vi "reprocess channel names for duplicates.vi"(11 "channels in":cluster{"Name":string, "Path":string}[](array[cluster])) -> (3 "processed channels":cluster{"Name":string, "Path":string}[](array[cluster]))   [LabVIEW 2026, in "Nominal Core Streaming Engine.lvlib"]
uses:
  Nominal Core Streaming Engine.lvlib
  <vilib>/Utility/miscctls.llb/LVMapReplaceAction.ctl
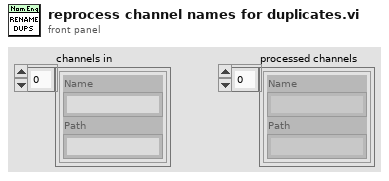
[diagram p1: front panel]
types:
  T1 = map{string, cluster{"original index":i32, "channel data":cluster{"Name":string, "Path":string}}[]}
  T2 = typedef "LVMapReplaceAction.ctl" = enum32{"Modify Entry only if found", "Add or Modify Entry", "Delete Entry"}
  T3 = cluster{"original index":i32, "channel data":cluster{"Name":string, "Path":string}}[]
  T4 = cluster{i32, cluster{"Name":string, "Path":string}}
  T5 = cluster{"original index":i32, "channel data":cluster{"Name":string, "Path":string}}
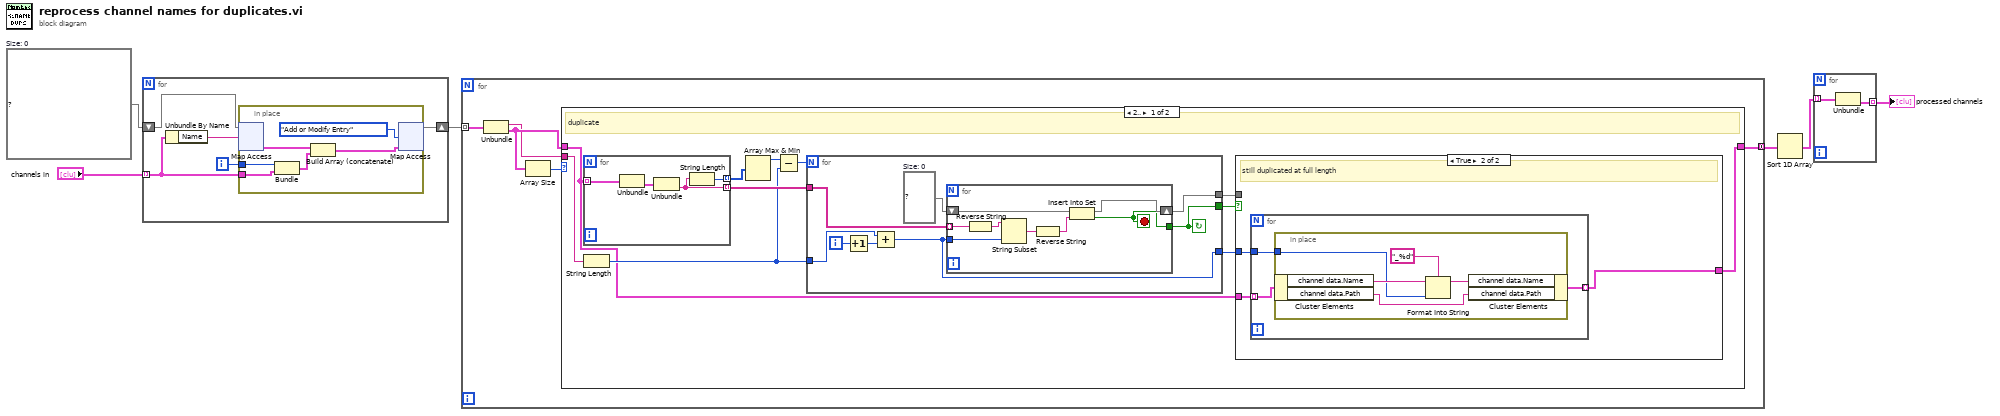
[diagram p0: block diagram]
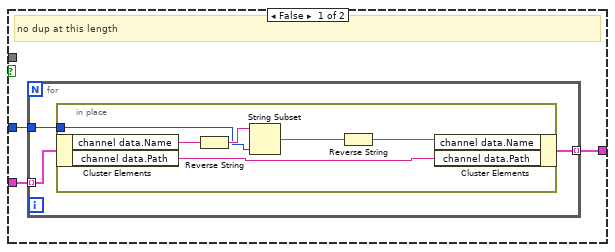
[diagram p2: hidden frame]
diagram:
  w5 = T1 {}  # Size: 0
  n1 = for {
    tunnel: "channels in" -> [w10] mode=indexing
    shift-right: [w8] -> w4
    shift-left: w5 -> [w9]
    i -> [w11]
    n2 = Unbundle By Name(w10) -> ("Name"=w7:string)
    n3 = in-place {
      in-place-border: w11 -> [w17]
      in-place-border: w10 -> [w16]
      n4 = in-place-map #1(w9, w7) -> (w13:T3)  [unwired: 1 in, 1 out]
      n5 = Bundle(w17, w16) -> (w14:T4)  [unwired: 1 in]
      n6 = Build Array (concatenate)(w13, w14) -> (w12:T3)
      n7 = in-place-map #1(w12, LVMapReplaceAction."Add or Modify Entry" ("action")) -> (w8:T1)  [unwired: 2 out]
    }
  }
  n8 = for {
    tunnel: w4 -> [w22] mode=indexing
    tunnel: [w19] -> w3 mode=concatenating
    n9 = Unbundle(w22) -> ("Name"=w18:string, w20:T3)
    n10 = Array Size(array=w20) -> (size(s)=w21:i32)
    n11 = case shown="2.." w21 {
      tunnel: w20 -> [w26 w77]
      tunnel: [w25 w77] -> w19
      tunnel: w18 -> [w32 _]
      frame 2.. {
        # "duplicate"
        n12 = for {
          tunnel: w26 -> [w76] mode=indexing
          tunnel: [w74] -> w33 mode=indexing
          tunnel: [w73] -> w31 mode=indexing
          n13 = Unbundle(w76) -> ("channel data"=w75:cluster{"Name":string, "Path":string})  [unwired: 1 out]
          n14 = Unbundle(w75) -> ("Path"=w74:string)  [unwired: 1 out]
          n15 = String Length(string=w74) -> (length=w73:i32)
        }
        n16 = String Length(string=w32) -> (length=w29:i32)
        n17 = Array Max & Min(array=w31) -> (max value=w30:i32)  [unwired: 3 out]
        n18 = Subtract(x=w30, y=w29) -> (x-y=w28:i32)
        n19 = for {
          N: w28 -> [_]
          tunnel: w33 -> [w61]
          tunnel: w29 -> [w63]
          tunnel: [w59] -> w27
          tunnel: [w58] -> w24
          tunnel: [w57] -> w23
          i -> [w64]
          stop <- w59 continue-if-true
          w60 = set{string} {}  # Size: 0
          n20 = Increment(x=w64) -> (x+1=w62:i32)
          n21 = Add(x=w63, y=w62) -> (x+y=w57:i32)
          n22 = for {
            tunnel: w61 -> [w72] mode=indexing
            tunnel: w57 -> [w70]
            shift-right: [w68] -> w58
            shift-left: w60 -> [w67]
            tunnel: [w66] -> w59
            stop <- w66 stop-if-true
            n23 = Reverse String(1:w72) -> (0:w71:string)
            n24 = String Subset(string=w71, length (rest)=w70) -> (substring=w69:string)  [unwired: 1 in]
            n25 = Reverse String(1:w69) -> (0:w65:string)
            n26 = Insert Into Set(10:w65, 11:w67) -> (2:w66:bool, 3:w68:set{string})
          }
        }
        n27 = case shown="True" w27 {
          tunnel: w26 -> [w36 w48]
          tunnel: [w35 w47] -> w25
          tunnel: w24 -> [_ _]
          tunnel: w23 -> [w34 w46]
          frame False {
            # "no dup at this length"
            n28 = for {
              tunnel: w36 -> [w39] mode=indexing
              tunnel: [w38] -> w35 mode=indexing
              tunnel: w34 -> [w37]
              n29 = in-place {
                in-place-border: w37 -> [w42]
                n30 = in-place-cluster #2(w39) -> ("channel data.Name"=w41:string, "channel data.Path"=w45:string)
                n31 = Reverse String(1:w41) -> (0:w43:string)
                n32 = String Subset(string=w43, length (rest)=w42) -> (substring=w44:string)  [unwired: 1 in]
                n33 = Reverse String(1:w44) -> (0:w40:string)
                n34 = in-place-cluster #2("channel data.Name"=w40, "channel data.Path"=w45) -> (w38:T5)
              }
            }
          }
          frame True {
            # "still duplicated at full length"
            n35 = for {
              tunnel: w48 -> [w51] mode=indexing
              tunnel: [w50] -> w47 mode=indexing
              tunnel: w46 -> [w49]
              n36 = in-place {
                in-place-border: w49 -> [w54]
                n37 = in-place-cluster #3(w51) -> ("channel data.Name"=w55:string, "channel data.Path"=w56:string)
                n38 = Format Into String(format string="_%d", initial string=w55, w54) -> (resulting string=w53:string)  [unwired: 1 in, 1 out]
                n39 = in-place-cluster #3("channel data.Name"=w53, "channel data.Path"=w56) -> (w50:T5)
              }
            }
          }
        }
      }
      frame ..1 {
      }
    }
  }
  n40 = Sort 1D Array(array=w3) -> (sorted array=w2:T3)
  n41 = for {
    tunnel: w2 -> [w79] mode=indexing
    tunnel: [w78] -> w1 mode=indexing
    n42 = Unbundle(w79) -> ("channel data"=w78:cluster{"Name":string, "Path":string})  [unwired: 1 out]
  }
  "processed channels" <- w1
